vi "更新线段.vi"(0 "参数":T1) -> ()   [LabVIEW 2020]
uses:
  Global variable.vi
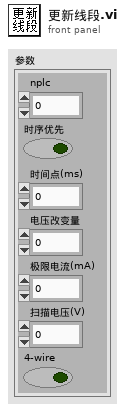
[diagram p1: front panel]
types:
  T1 = cluster{"nplc":dbl, "时序优先":bool, "时间点(ms)":dbl, "电压改变量":dbl, "极限电流(mA)":dbl, "扫描电压(V)":dbl, "4-wire ":bool}
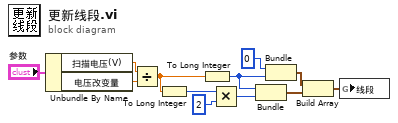
[diagram p0: block diagram]
diagram:
  n1 = Unbundle By Name("参数") -> ("扫描电压(V)"=w5:dbl, "电压改变量"=w6:dbl)
  n2 = Divide(x=w5, y=w6) -> (x/y=w9:dbl)
  n3 = To Long Integer(number=w9) -> (32bit integer=w10:i32)
  n4 = To Long Integer(number=w9) -> (32bit integer=w11:i32)
  n5 = Multiply(x=w10, y=2) -> (x*y=w12:i32)
  n6 = Bundle(w11, w12) -> (w8:cluster{i32, i32})  [unwired: 1 in]
  n7 = Bundle(0, w11) -> (w7:cluster{i32, i32})  [unwired: 1 in]
  n8 = Build Array(w7, w8) -> (w2:cluster{i32, i32}[])
  n9 = global write "Global variable.vi" "线段"(w2) -> ()
